vi "AdminLogInAddMoreTrials.vi"() -> ()   [LabVIEW 2013]
uses:
  <vilib>/addons/database/Connection.llb/DB Tools Open Connec (String).vi
  <vilib>/addons/database/_DB Variant To Data/Database Variant To Data.xnode
  <vilib>/addons/database/NI_Database_API.lvlib
panel:
  in  "Attempts":dbl=5.0
  out "AdminNo.Accepted?":string
  in  "Student Admin No:":string
  in  "Confirm&Back":bool
  # "PLease Enter how many more Attempts for which Student.\n(The default value is 5 trials)"
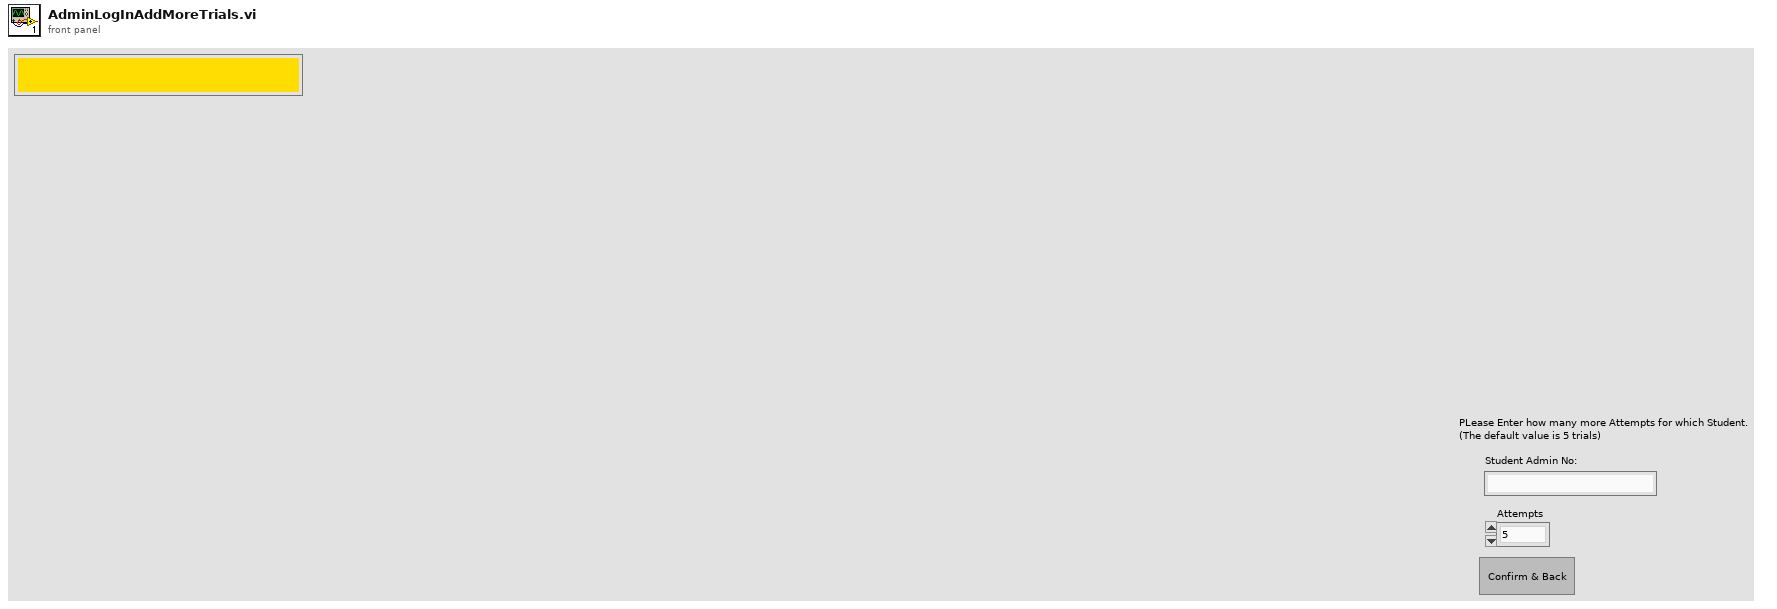
[diagram p1: front panel]
types:
  T1 = typedef "NI_Database_API.lvlib/Conn ObjectReference.ctl" = refnum<k1>
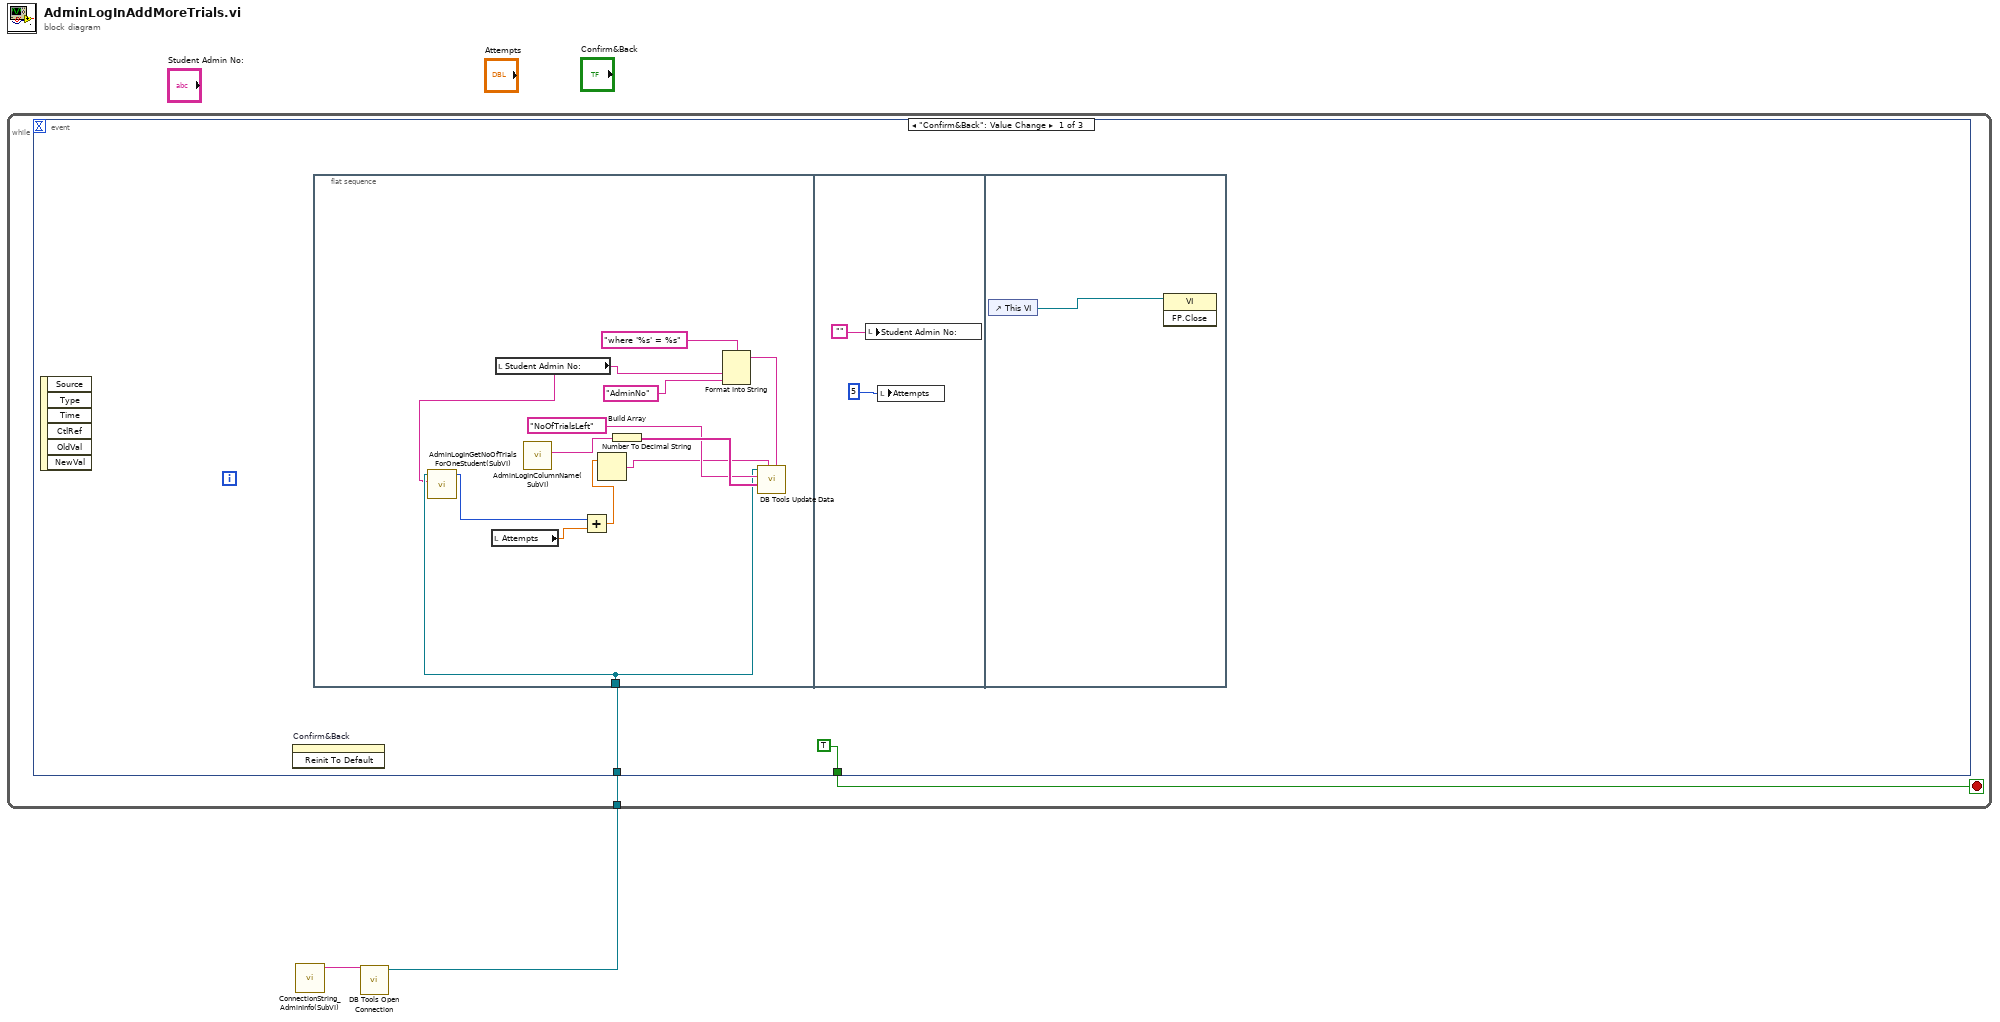
[diagram p0: block diagram]
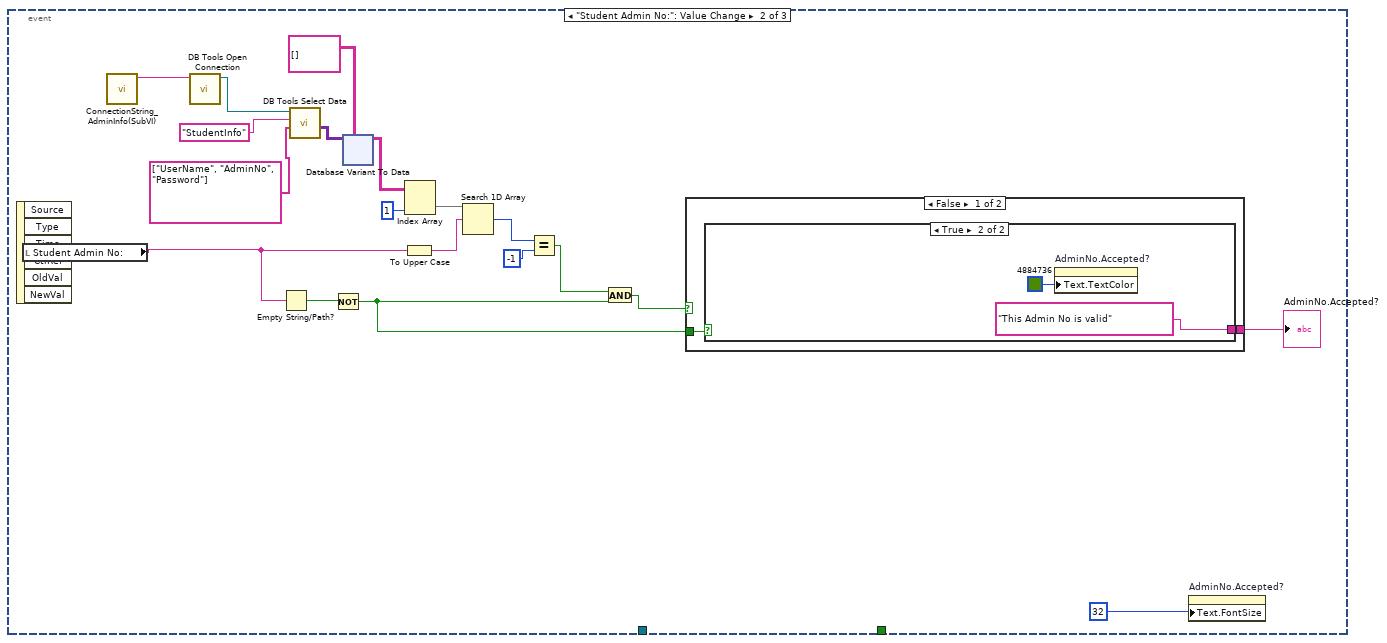
[diagram p2: hidden frame]
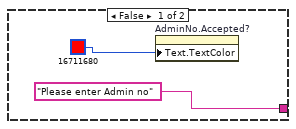
[diagram p3: hidden frame]
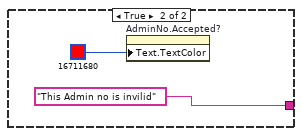
[diagram p4: hidden frame]
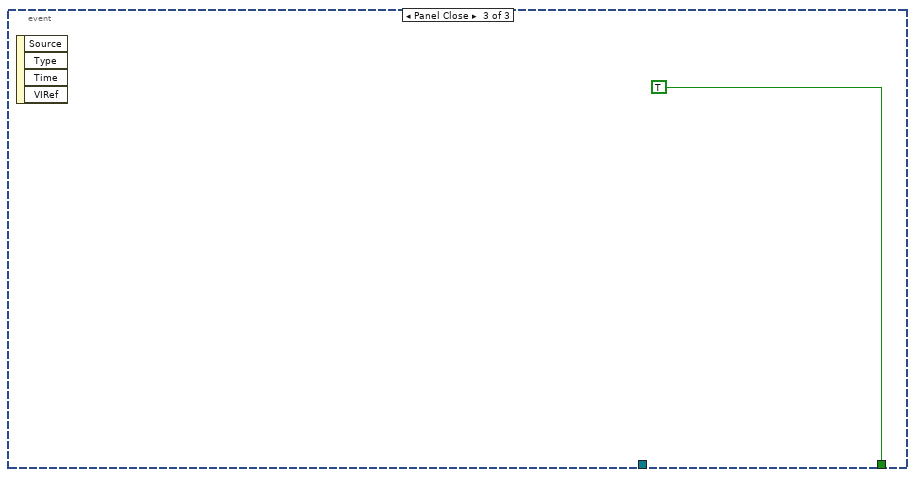
[diagram p5: hidden frame]
diagram:
  n1 = call "ConnectionString_AdminInfo(SubVI).vi"() -> ("ConnectionString"=w2:string)  [unwired: 11 in]
  n2 = call-poly <vilib>:"DB Tools Open Connection.vi"("connection information"=w2) -> ("connection reference"=w1:T1)  [unwired: 7 in, 1 out]
  n3 = while {
    tunnel: w1 -> [w3]
    stop <- w4 stop-if-true
    n4 = event shown="[0] \"Confirm&Back\": Value Change" {
      selector: _ -> [_ _ _]
      dyn-events: _ -> [_ _ _]
      timeout: _ -> [_ _ _]
      tunnel: [TRUE _ TRUE] -> w4
      tunnel: w3 -> [w5 _ _]
      event "Confirm&Back": Value Change {
        n5 = event-data() -> ()  [unwired: 1 in, 6 out]
        n6 = invoke on="Confirm&Back" class="Bool (strict)" method="Reinit To Default"() -> ()  [unwired: 3 in, 3 out]
        n7 = flat-sequence {
          tunnel: w5 -> [w9]
          frame #0 {
            n8 = local read "Attempts"() -> (w12:dbl)
            n9 = local read "Student Admin No:"() -> (w8:string)
            n10 = call "AdminLogInGetNoOfTrialsForOneStudent(SubVI).vi"("Admin no"=w8, "Refnum in"=w9) -> ("NoOfTrials"=w7:i32)  [unwired: 9 in]
            n11 = call "AdminLogInColumnName(SubVI).vi"() -> ("Path for Score Table"=w10:string)  [unwired: 11 in]
            n12 = Add(x=w7, y=w12) -> (x+y=w11:dbl)
            n13 = Number To Decimal String(number=w11) -> (decimal integer string=w13:string)  [unwired: 1 in]
            n14 = Build Array(w10) -> (w15:string[])
            n15 = Format Into String(format string="where '%s' = %s", w8, "AdminNo") -> (resulting string=w18:string)  [unwired: 2 in, 1 out]
            n16 = call <vilib>:"DB Tools Update Data.vi"("condition"=w18, "data"=w13, "columns"=w15, "table"="NoOfTrialsLeft", "connection reference"=w9) -> ()  [unwired: 5 in, 2 out]
          }
          frame #1 {
            n17 = local write "Student Admin No:"("") -> ()
            n18 = local write "Attempts"(5) -> ()
          }
          frame #2 {
            n19 = control-ref of="This VI"() -> (w21:refnum<vi>)
            n20 = invoke class="VI" method="FP.Close"(reference=w21) -> ()  [unwired: 2 in, 3 out]
          }
        }
      }
      event "Student Admin No:": Value Change {
        n21 = event-data() -> ()  [unwired: 1 in, 6 out]
        n22 = local read "Student Admin No:"() -> (w23:string)
        n23 = call "ConnectionString_AdminInfo(SubVI).vi"() -> ("ConnectionString"=w38:string)  [unwired: 11 in]
        n24 = call-poly <vilib>:"DB Tools Open Connection.vi"("connection information"=w38) -> ("connection reference"=w39:T1)  [unwired: 7 in, 1 out]
        n25 = Empty String/Path?(string/path=w23) -> (empty?=w33:bool)
        n26 = call <vilib>:"DB Tools Select Data.vi"("columns"=string[] ["UserName", "AdminNo", "Password"], "table"="StudentInfo", "connection reference"=w39) -> ("data"=w26:variant[][])  [unwired: 3 in, 2 out]
        n27 = Not(x=w33) -> (.not. x?=w35:bool)
        n28 = xnode "Database Variant To Data"("database variant"=w26, "type"=string[][] []) -> ("data"=w27:string[][])  [unwired: 1 in, 1 out]
        n29 = To Upper Case(1:w23) -> (0:w30:string)
        n30 = Index Array(array=w27, index (col)=1) -> (element=w29:string[])  [unwired: 1 in]
        n31 = Search 1D Array(1D array=w29, element=w30) -> (index of element=w31:i32)  [unwired: 1 in]
        n32 = Equal?(x=w31, y=-1) -> (x = y?=w34:bool)
        n33 = And(x=w34, y=w35) -> (x .and. y?=w40:bool)
        n34 = case shown="False" w40 {
          tunnel: w35 -> [w41 _]
          tunnel: [w42 "This Admin no is invilid"] -> w36
          frame False {
            n35 = case shown="True" w41 {
              tunnel: ["Please enter Admin no" "This Admin No is valid"] -> w42
              frame False {
                n36 = property on="AdminNo.Accepted?" class="Str"("Text.TextColor"=u32 16711680) -> ()  [unwired: 2 in, 2 out]
              }
              frame True {
                n37 = property on="AdminNo.Accepted?" class="Str"("Text.TextColor"=u32 4884736) -> ()  [unwired: 2 in, 2 out]
              }
            }
          }
          frame True {
            n38 = property on="AdminNo.Accepted?" class="Str"("Text.TextColor"=u32 16711680) -> ()  [unwired: 2 in, 2 out]
          }
        }
        "AdminNo.Accepted?" <- w36
        n39 = property on="AdminNo.Accepted?" class="Str"("Text.FontSize"=32) -> ()  [unwired: 2 in, 2 out]
      }
      event Panel Close {
        n40 = event-data() -> ()  [unwired: 1 in, 4 out]
      }
    }
  }
